vi "Normalizer32_nr.vi"(4 "x":u32 format="%032b") -> (1 "normalized":u32, 2 "shift":i8)   [LabVIEW 2010]
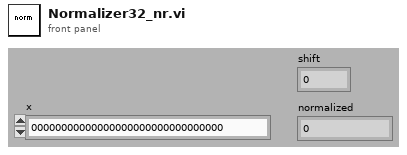
[diagram p1: front panel]
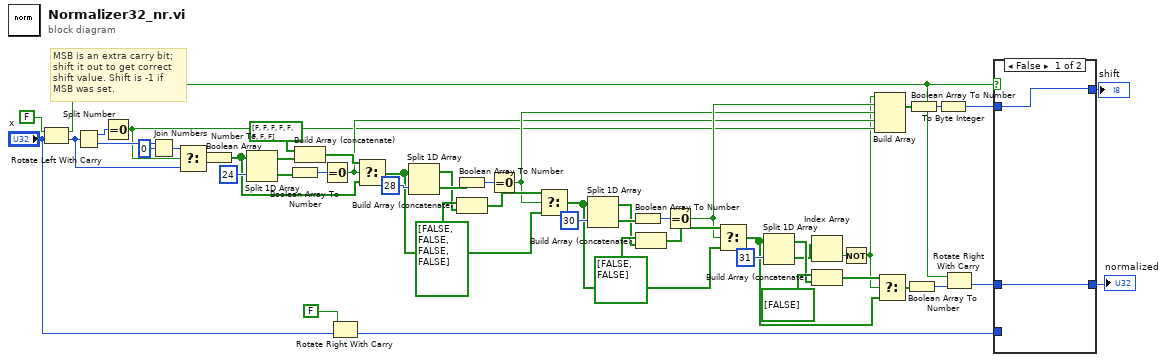
[diagram p0: block diagram]
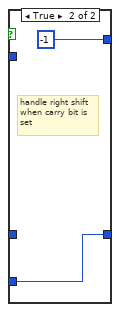
[diagram p2: hidden frame]
diagram:
  # "MSB is an extra carry bit; shift it out to get correct shift value. Shift is -1 if MSB was set."
  n1 = Rotate Left With Carry(2:"x", 3:FALSE ("carry")) -> (0:w13:u32, 1:w8:bool)
  n2 = Split Number(x=w13) -> (hi(x)=w51:u16, lo(x)=w52:u16)
  n3 = Equal To 0?(x=w51) -> (x = 0?=w17:bool)
  n4 = Join Numbers(hi=w52, lo=u16 0) -> ((hi.lo)=w50:u32)
  n5 = Select(t=w50, s=w17, f=w13) -> (s? t:f=w48:u32)
  n6 = Number To Boolean Array(number=w48) -> (Boolean array=w43:bool[])
  n7 = Split 1D Array(array=w43, index=24) -> (first subarray=w26:bool[], second subarray=w27:bool[])
  n8 = Boolean Array To Number(Boolean array=w27) -> (number=w46:u8)
  n9 = Build Array (concatenate)(bool[] [FALSE, FALSE, FALSE, FALSE, FALSE, FALSE, FALSE, FALSE], w26) -> (w44:bool[])
  n10 = Equal To 0?(x=w46) -> (x = 0?=w18:bool)
  n11 = Rotate Right With Carry(2:"x", 3:FALSE ("carry")) -> (0:w1:u32)  [unwired: 1 out]
  n12 = Select(t=w44, s=w18, f=w43) -> (s? t:f=w38:bool[])
  n13 = Split 1D Array(array=w38, index=28) -> (first subarray=w24:bool[], second subarray=w25:bool[])
  n14 = Boolean Array To Number(Boolean array=w25) -> (number=w40:u8)
  n15 = Build Array (concatenate)(bool[] [FALSE, FALSE, FALSE, FALSE], w24) -> (w42:bool[])
  n16 = Equal To 0?(x=w40) -> (x = 0?=w19:bool)
  n17 = Select(t=w42, s=w19, f=w38) -> (s? t:f=w34:bool[])
  n18 = Split 1D Array(array=w34, index=30) -> (first subarray=w22:bool[], second subarray=w23:bool[])
  n19 = Boolean Array To Number(Boolean array=w23) -> (number=w33:u8)
  n20 = Build Array (concatenate)(bool[] [FALSE, FALSE], w22) -> (w35:bool[])
  n21 = Equal To 0?(x=w33) -> (x = 0?=w20:bool)
  n22 = Select(t=w35, s=w20, f=w34) -> (s? t:f=w29:bool[])
  n23 = Split 1D Array(array=w29, index=31) -> (first subarray=w21:bool[], second subarray=w16:bool[])
  n24 = Index Array(array=w16) -> (element=w15:bool)  [unwired: 1 in]
  n25 = Build Array (concatenate)(bool[] [FALSE], w21) -> (w32:bool[])
  n26 = Not(x=w15) -> (.not. x?=w14:bool)
  n27 = Build Array(w14, w20, w19, w18, w17) -> (w11:bool[])
  n28 = Select(t=w32, s=w14, f=w29) -> (s? t:f=w28:bool[])
  n29 = Boolean Array To Number(Boolean array=w28) -> (number=w9:u32)
  n30 = Boolean Array To Number(Boolean array=w11) -> (number=w10:u8)
  n31 = To Byte Integer(number=w10) -> (8bit integer=w6:i8)
  n32 = Rotate Right With Carry(2:w9, 3:w8) -> (0:w5:u32)  [unwired: 1 out]
  n33 = case shown="False" w8 {
    tunnel: [w54 i8 -1 ("t")] -> w7
    tunnel: w6 -> [w54 _]
    tunnel: w5 -> [w53 _]
    tunnel: [w53 w55] -> w4
    tunnel: w1 -> [_ w55]
    frame False {
    }
    frame True {
      # "handle right shift\nwhen carry bit is\nset"
    }
  }
  "normalized" <- w4
  "shift" <- w7
